vi "GEN_TimerPerS.vi"(9 "Data_In":T1 {"GUI Data Cluster"."SBR" format="%08b"}, 10 "Config_In":T3={"General"={"Config.ini"=path "", "Default Logging Path"=path ""}, "Hardware"={"AHC VISA COM"="", "Measure Rate (1/s)"=0, "Global T VAR"="", "Global B VAR"=""}, "Operation"={"Operation Mode"=enum."Idle-Off", "Status"="", "NewLog?"=FALSE}}) -> (0 "Time":bool, 1 "Data_In 2":T1 {"GUI Data Cluster"."SBR" format="%08b"}, 2 "Config_In 2":T3={"General"={"Config.ini"=path "", "Default Logging Path"=path ""}, "Hardware"={"AHC VISA COM"="", "Measure Rate (1/s)"=0, "Global T VAR"="", "Global B VAR"=""}, "Operation"={"Operation Mode"=enum."Idle-Off", "Status"="", "NewLog?"=FALSE}})   [LabVIEW 2021]
uses:
  Data_Cluster.ctl
  Measurement_Cluster.ctl
  Config_Cluster.ctl
  Mode_Enum.ctl
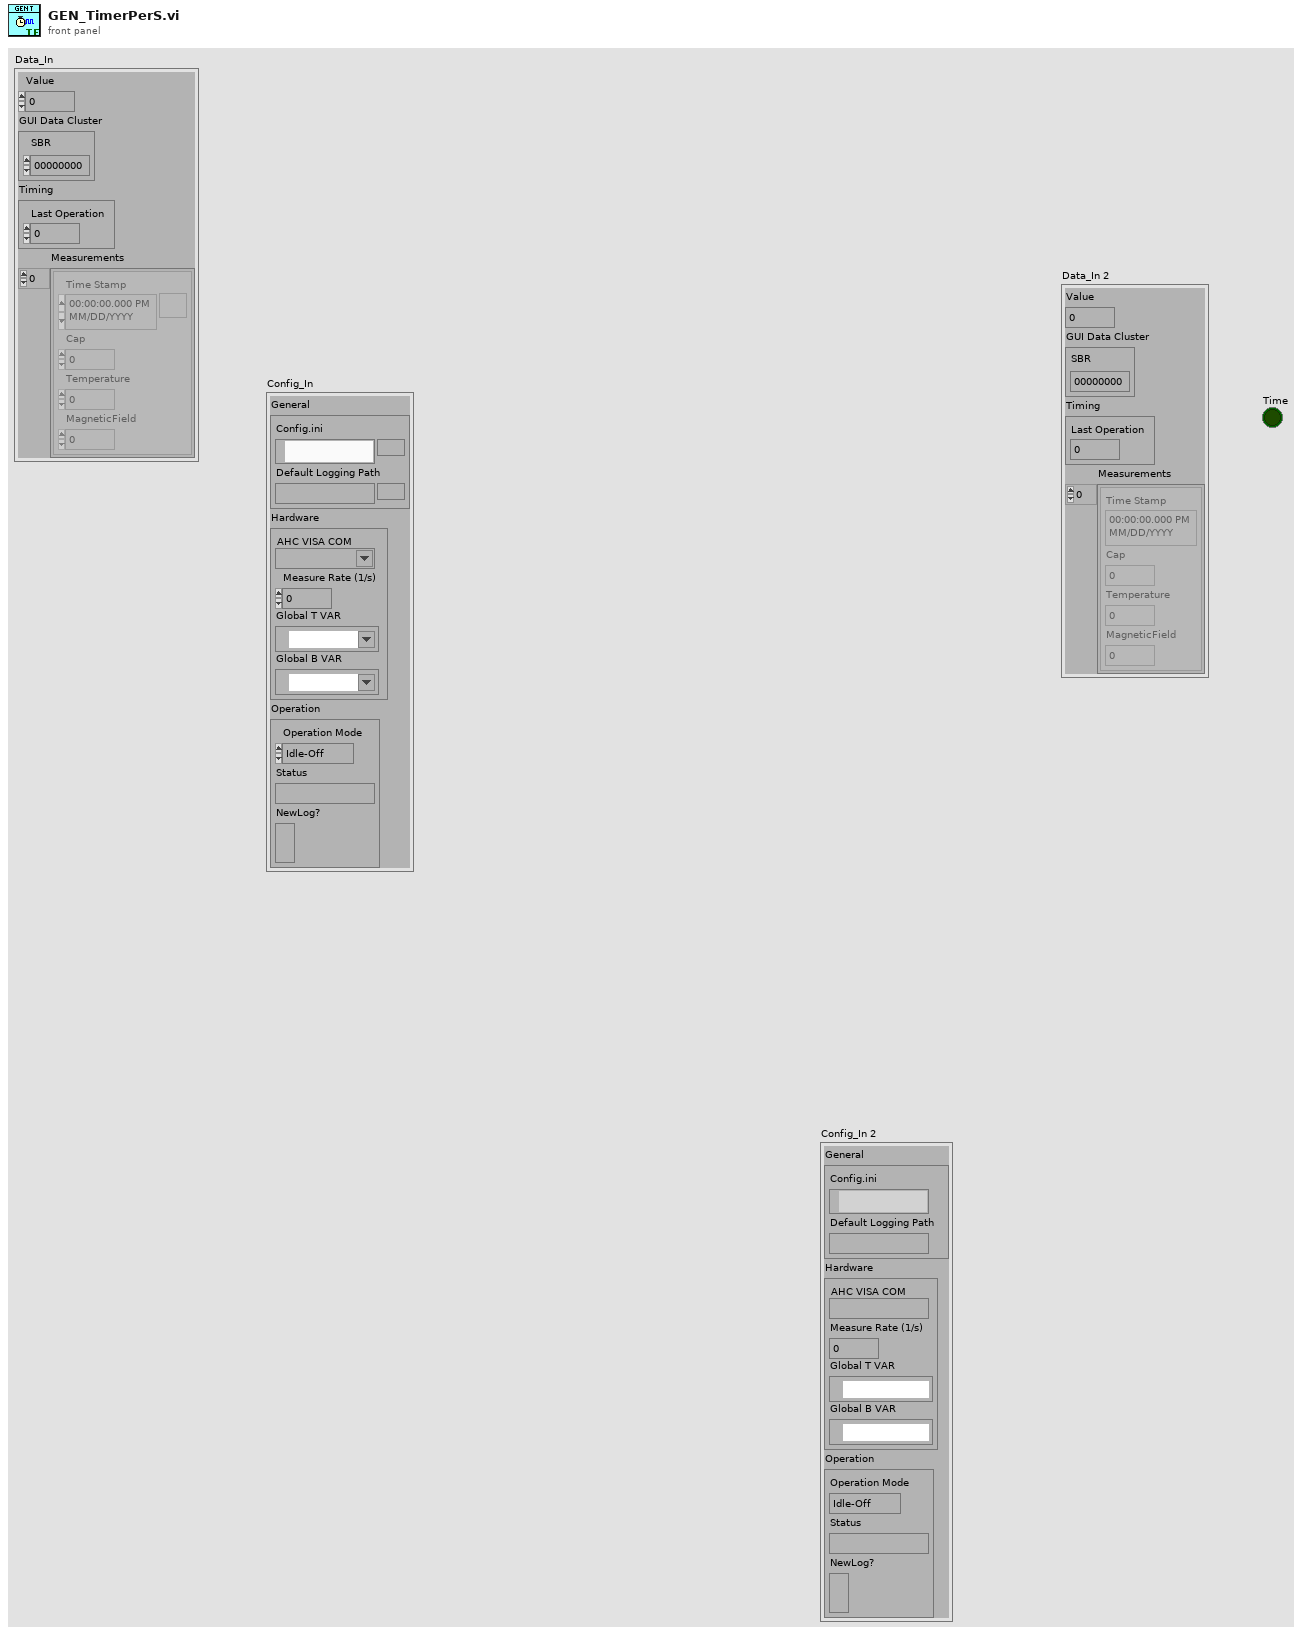
[diagram p1: front panel]
types:
  T1 = typedef "Data_Cluster.ctl" = cluster{"Value":dbl, "GUI Data Cluster":cluster{"SBR":u8}, "Timing":cluster{"Last Operation":dbl}, "Measurements":T2[]}
  T2 = typedef "Measurement_Cluster.ctl" = cluster{"Time Stamp":timestamp, "Cap":dbl, "Temperature":dbl, "MagneticField":dbl}
  T3 = typedef "Config_Cluster.ctl" = cluster{"General":cluster{"Config.ini":path, "Default Logging Path":path}, "Hardware":cluster{"AHC VISA COM":refnum<visa-resource-name>, "Measure Rate (1/s)":i32, "Global T VAR":refnum<k21>, "Global B VAR":refnum<k21>}, "Operation":cluster{"Operation Mode":T4, "Status":string, "NewLog?":bool}}
  T4 = typedef "Mode_Enum.ctl" = enum16{"Logging", "Idle-Off", "Idle"}
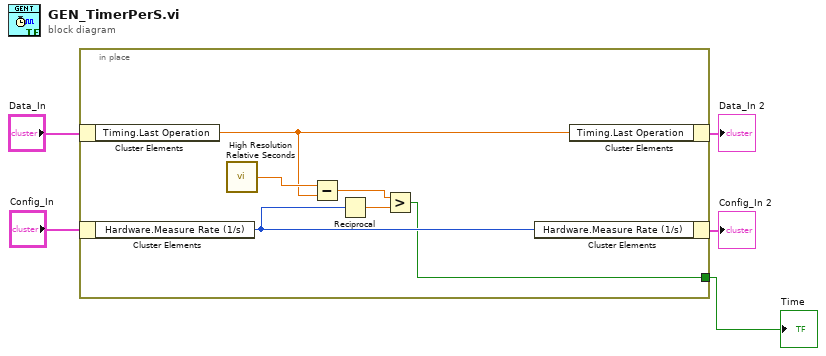
[diagram p0: block diagram]
diagram:
  n1 = in-place {
    in-place-border: [w6] -> w1
    n2 = in-place-cluster #1("Data_In") -> ("Timing.Last Operation"=w9:dbl)
    n3 = in-place-cluster #2("Config_In") -> ("Hardware.Measure Rate (1/s)"=w10:i32)
    n4 = call <vilib>:"High Resolution Relative Seconds.vi"() -> ("relative seconds"=w11:dbl)
    n5 = Subtract(x=w11, y=w9) -> (x-y=w7:dbl)
    n6 = Reciprocal(x=w10) -> (1/x=w8:dbl)
    n7 = Greater?(x=w7, y=w8) -> (0:w6:bool)
    n8 = in-place-cluster #2("Hardware.Measure Rate (1/s)"=w10) -> (→"Config_In 2":T3)
    n9 = in-place-cluster #1("Timing.Last Operation"=w9) -> (→"Data_In 2":T1)
  }
  "Time" <- w1
